vi "get country index from config.vi"(7 "Countries":string[](array[string]), 8 "error in (no error)":errorcluster, 9 "key":string, 10 "Section":string, 11 "Refnum in":T1) -> (0 "error out":errorcluster, 2 "index of element":i32, 3 "Refnum out":T1)   [LabVIEW 2019]
uses:
  <vilib>/Utility/config.llb/Config Data RefNum.ctl
  <vilib>/Utility/config.llb/Read Key (String).vi
  <vilib>/Utility/config.llb/Write Key (String).vi
  <vilib>/Utility/config.llb/NI_LVConfig.lvlib
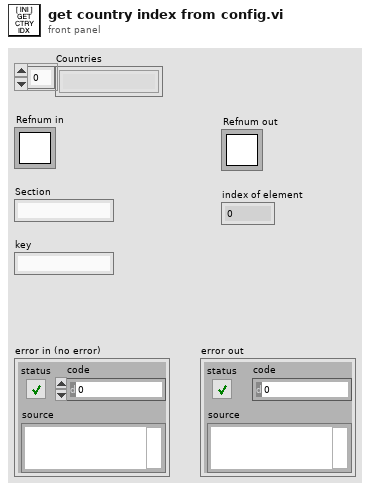
[diagram p1: front panel]
types:
  T1 = typedef "NI_LVConfig.lvlib/Config Data RefNum.ctl" = refnum<k1>
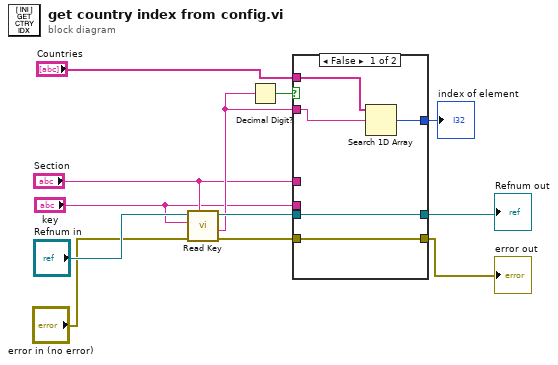
[diagram p0: block diagram]
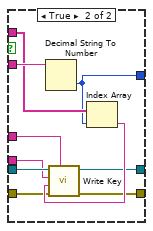
[diagram p2: hidden frame]
diagram:
  n1 = call-poly <vilib>:"Read Key.vi"("section"="Section", "error in (no error)"="error in (no error)", "key"="key", "refnum"="Refnum in") -> ("error out"=w4:errorcluster, "value"=w3:string, "refnum out"=w6:T1)  [unwired: 4 in, 1 out]
  n2 = Decimal Digit?(1:w3) -> (0:w8:bool)
  n3 = case shown="False" w8 {
    tunnel: w3 -> [w17 w27]
    tunnel: [w15 w22] -> w12
    tunnel: "Countries" -> [w16 w23]
    tunnel: w6 -> [w14 w26]
    tunnel: "Section" -> [_ w25]
    tunnel: "key" -> [_ w24]
    tunnel: [w14 w20] -> w10
    tunnel: w4 -> [w13 w19]
    tunnel: [w13 w18] -> w11
    frame False {
      n4 = Search 1D Array(1D array=w16, element=w17) -> (index of element=w15:i32)  [unwired: 1 in]
    }
    frame True {
      n5 = Decimal String To Number(string=w27) -> (number=w22:i32)  [unwired: 2 in, 1 out]
      n6 = Index Array(array=w23, index=w22) -> (element=w21:string)
      n7 = call-poly <vilib>:"Write Key.vi"("section"=w25, "error in (no error)"=w19, "value"=w21, "key"=w24, "refnum"=w26) -> ("error out"=w18:errorcluster, "refnum out"=w20:T1)  [unwired: 4 in, 1 out]
    }
  }
  "index of element" <- w12
  "error out" <- w11
  "Refnum out" <- w10
